vi "AAA Charger Test Set Catalog.vi"   [LabVIEW 2010]
uses:
  Charger/Charger_States_Control.ctl
  Charger_Input Control.ctl
panel:
  # "Charger Test Set Catalog"
types:
  T1 = typedef "Charger_Input Control.ctl" = cluster{"address":refnum<visa-resource-name>, "position":i32, "setpoint":dbl}
  T2 = typedef "Charger_States_Control.ctl" = enum16{"Enable", "Disable", "Adjust", "Pause", "na"}
  T3 = enum16{"Disable", "Enable", "Update", "Get Info"}
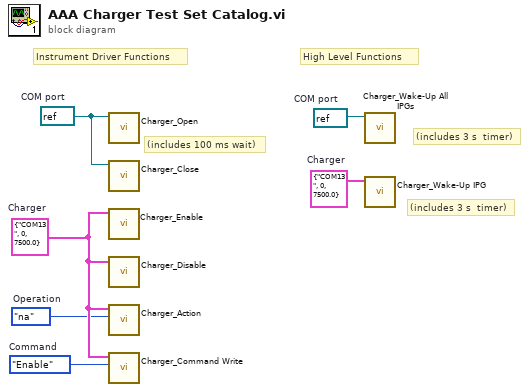
[diagram p0: block diagram]
diagram:
  w1 = refnum<visa-resource-name> refnum  # COM port
  w2 = T1 {"address"="COM13", "position"=0, "setpoint"=7500.0}  # Charger
  w3 = Charger_States_Control."na"  # Operation
  w4 = refnum<visa-resource-name> refnum  # COM port
  w5 = T1 {"address"="COM13", "position"=0, "setpoint"=7500.0}  # Charger
  w6 = T3."Enable"  # Command
  # "(includes 3 s  timer)"
  # "(includes 100 ms wait)"
  # "(includes 3 s  timer)"
  # "High Level Functions"
  # "Instrument Driver Functions"
  n1 = call "Charger_Open.vi"("Charger COM port"=w4) -> ()  [unwired: 6 in, 1 out]
  n2 = call "Charger_Close.vi"("address"=w4) -> ()  [unwired: 6 in, 1 out]
  n3 = call "Charger_Enable.vi"("Charger"=w5) -> ()  [unwired: 8 in, 1 out]
  n4 = call "Charger_Disable.vi"("Charger"=w5) -> ()  [unwired: 8 in, 1 out]
  n5 = call "Charger_Action.vi"("Operation"=w3, "Charger"=w5) -> ()  [unwired: 7 in, 1 out]
  n6 = call "Charger_Command Write.vi"("Command"=w6, "Charger"=w5) -> ()  [unwired: 6 in, 2 out]
  n7 = call "Charger_Wake-Up All IPGs.vi"("Charger COM Port"=w1) -> ()  [unwired: 10 in, 1 out]
  n8 = call "Charger_Wake-Up IPG.vi"("Charger"=w2) -> ()  [unwired: 8 in, 1 out]
